vi "strings to line.vi"(11 "strings":string[](array[string])) -> (3 "line":T1)   [LabVIEW 2013, in "Modbus Module editor node.lvclass"]
doc: "Platypus Framework 1.0.1.65\nNI Systems Engineering - National Instruments"
uses:
  Modbus Module editor node.lvclass
  table line.ctl
  module/module channel/Modbus Module Channel.lvclass
  <vilib>/NI/Tag Bus/tag/Data Type.ctl
  permissions.ctl
  <vilib>/NI/Tag Bus/tag/tag descriptor.lvclass/tag descriptor.ctl
  <vilib>/NI/Tag Bus Module Framework/channel/TBM channel.lvclass/TBM channel.ctl
  <vilib>/NI/Tag Bus/tag/write tag name.vi
  <vilib>/NI/Tag Bus Module Framework/channel/Write channel classification.vi
  <vilib>/NI/Tag Bus/tag/write data type.vi
  <vilib>/NI/Tag Bus/tag/tag descriptor.lvclass
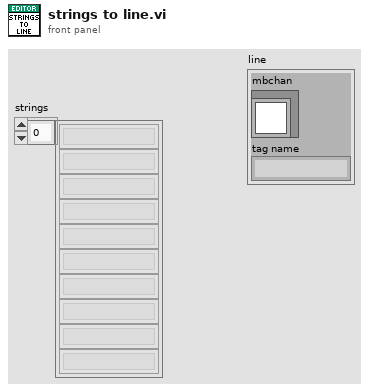
[diagram p1: front panel]
types:
  T1 = typedef "Modbus Module editor node.lvclass/table line.ctl" = cluster{"mbchan":refnum<class "Modbus Module Channel.lvclass">, "tag name":string}
  T2 = typedef "Modbus Module editor node.lvclass/permissions.ctl" = enum32{"Read from MB", "Write to MB"}
  T3 = typedef "tag bus.lvlib/tag descriptor.lvclass/Data Type.ctl" = enum16{"Double", "Single", "I64", "I32", "I16", "I8", "U64", "U32", "U16", "U8", "Boolean", "String", "Array of Double", "Array of Single", "Array of I64", "Array of I32", "Array of I16", "Array of I8", "Array of U64", "Array of U32", "Array of U16", "Array of U8", "Array of Boolean", "Array of String"}
  T4 = typedef "TBM channel.lvclass/channel classification.ctl" = enum16{"input data", "output data", "processing parameter", "processing result"}
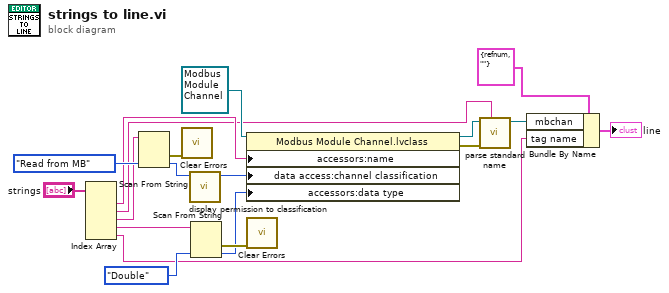
[diagram p0: block diagram]
diagram:
  n1 = Index Array(array="strings") -> (element #1=w8:string, element #2=w4:string, element #3=w3:string, element #4=w2:string, element #5=w1:string)  [unwired: 5 in]
  n2 = Scan From String(input string=w3, default 1=permissions."Read from MB" ("direction")) -> (error out=w14:errorcluster, output 1=w12:T2)  [unwired: 3 in, 2 out]
  n3 = call <vilib>:"Clear Errors.vi"("error in (no error)"=w14) -> ()  [unwired: 6 in, 1 out]
  n4 = call "display permission to classification.vi"("display permissions"=w12) -> ("channel classification"=w9:T4)  [unwired: 10 in]
  n5 = Scan From String(input string=w2, default 1=Data_Type."Double" ("data type")) -> (error out=w16:errorcluster, output 1=w10:T3)  [unwired: 3 in, 2 out]
  n6 = property class="Modbus Module Channel.lvclass"(reference=refnum<class "Modbus Module Channel.lvclass"> refnum ("Modbus Module Channel"), "accessors:name"=w8, "data access:channel classification"=w9, "accessors:data type"=w10) -> (reference out=w7:refnum<class "Modbus Module Channel.lvclass">, error out=w6:errorcluster)  [unwired: 1 in]
  n7 = call <vilib>:"Clear Errors.vi"("error in (no error)"=w16) -> ()  [unwired: 6 in, 1 out]
  n8 = call "parse standard name.vi"("standard name"=w4, "error in"=w6, "Modbus Module Channel in"=w7) -> ("Modbus Module Channel out"=w5:refnum<class "Modbus Module Channel.lvclass">)  [unwired: 7 in, 1 out]
  n9 = Bundle By Name(cluster=T1 {"mbchan"=refnum, "tag name"=""} ("line"), "mbchan"=w5, "tag name"=w1) -> (→"line":T1)
